vi "GlobalConstReceiverPort.vi"() -> (1 "receiver port (0)":u16)   [LabVIEW 2019, in "Proccess.lvclass"]
uses:
  Proccess.lvclass
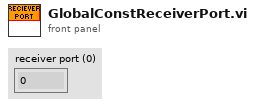
[diagram p1: front panel]
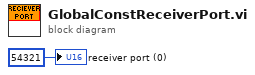
[diagram p0: block diagram]
diagram:
  "receiver port (0)" <- u16 54321 ("receiver port (0)")
